vi "Write Sensitivity(x).vi"(8 "error in (no error)":errorcluster, 10 "Sensitivity(x)":dbl, 11 "Joysticks in":refnum<class "Joysticks.lvclass">) -> (0 "error out":errorcluster, 3 "Joysticks out":refnum<class "Joysticks.lvclass">)   [LabVIEW 2019, in "Joysticks.lvlib" / "Joysticks.lvclass"]
uses:
  Joysticks.lvclass
  Joysticks.lvclass/Joysticks.ctl
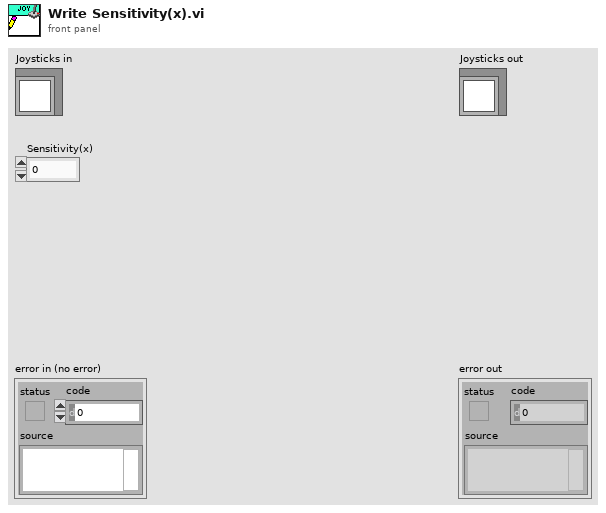
[diagram p1: front panel]
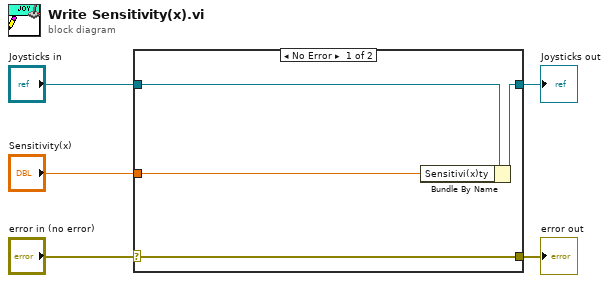
[diagram p0: block diagram]
diagram:
  n1 = case shown="No Error" "error in (no error)" {
    selector: "error in (no error)" -> [w9 w10]
    tunnel: [w9 w10] -> w4
    tunnel: [w7 w11] -> w2
    tunnel: "Joysticks in" -> [w8 w11]
    tunnel: "Sensitivity(x)" -> [w6 _]
    frame No Error {
      n2 = Bundle By Name(cluster=w8, "Sensitivi(x)ty"=w6) -> (w7:refnum<class "Joysticks.lvclass">)
    }
    frame Error {
    }
  }
  "error out" <- w4
  "Joysticks out" <- w2
